vi "Direction Detection Algorithm.vi"(4 "Current Position":u16, 5 "State Data in":T1) -> (2 "State Data Out":T1)   [LabVIEW 2015, in "Engine Simulation Toolkit.lvlib" / "Directional Speed.lvlib"]
uses:
  Directional Speed.lvlib
  State Data.ctl
  Settings.ctl
  State.ctl
  Engine Simulation Toolkit.lvlib
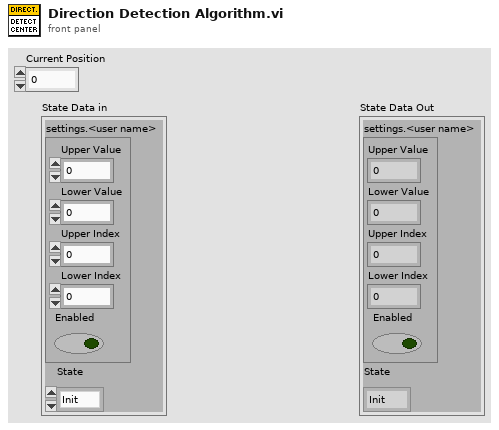
[diagram p1: front panel]
types:
  T1 = typedef "Engine Simulation Toolkit.lvlib/Directional Speed.lvlib/State Data.ctl" = cluster{"settings.<user name>":T2, "State":T3}
  T2 = typedef "Engine Simulation Toolkit.lvlib/Directional Speed.lvlib/Settings.ctl" = cluster{"Upper Value":u16, "Lower Value":u16, "Upper Index":fxp<+,10,10>, "Lower Index":fxp<+,10,10>, "Enabled":bool}
  T3 = typedef "Engine Simulation Toolkit.lvlib/Directional Speed.lvlib/State.ctl" = enum8{"Init", "Detect", "Positive Move td", "Negative Move td", "tf", "tr"}
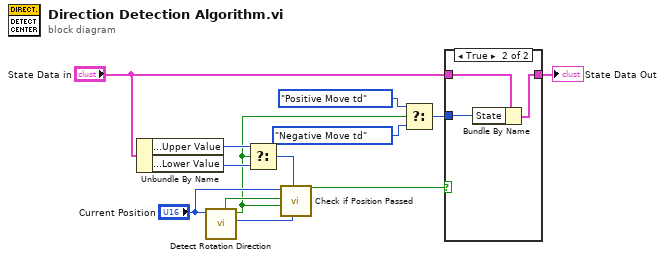
[diagram p0: block diagram]
diagram:
  n1 = Unbundle By Name("State Data in") -> ("settings.<user name>.Upper Value"=w8:u16, "settings.<user name>.Lower Value"=w7:u16)
  n2 = call "Detect Rotation Direction.vi"("position"="Current Position") -> ("previous position (n-1)"=w9:u16, "rotated forward or stopped"=w5:bool, "cycle wrapped"=w10:bool)  [unwired: 8 in]
  n3 = Select(t=w8, s=w5, f=w7) -> (s? t:f=w6:u16)
  n4 = call "Check if Position Passed.vi"("previous position (n-1)"=w9, "trigger position"=w6, "rotated forward"=w5, "cycle wrapped"=w10, "position"="Current Position") -> ("trigger"=w1:bool)  [unwired: 6 in]
  n5 = Select(t=State."Positive Move td", s=w5, f=State."Negative Move td" ("t")) -> (s? t:f=w2:T3)
  n6 = case shown="True" w1 {
    tunnel: [w14 w17] -> w13
    tunnel: "State Data in" -> [w14 w16]
    tunnel: w2 -> [_ w15]
    frame False {
    }
    frame True {
      n7 = Bundle By Name(cluster=w16, "State"=w15) -> (w17:T1)
    }
  }
  "State Data Out" <- w13
